vi "Placas_Foco.vi"() -> ()   [LabVIEW 2021]
uses:
  <vilib>/userDefined/High Color/IMAQdx.ctl
  <vilib>/vision/driver/NI_Vision_Acquisition_Software.lvlib
  <vilib>/vision/NI_Vision_Development_Module.lvlib
panel:
  out "String":string
  out "Matches[0].Position.y":sgl
  out "Matches[0].Position.x":sgl
  in  "Reconocer":bool
  in  "Stop":bool
  in  "Camara":T1
  out "Imagen":T2(plugin-control)
  out "Muestra":T2(plugin-control)
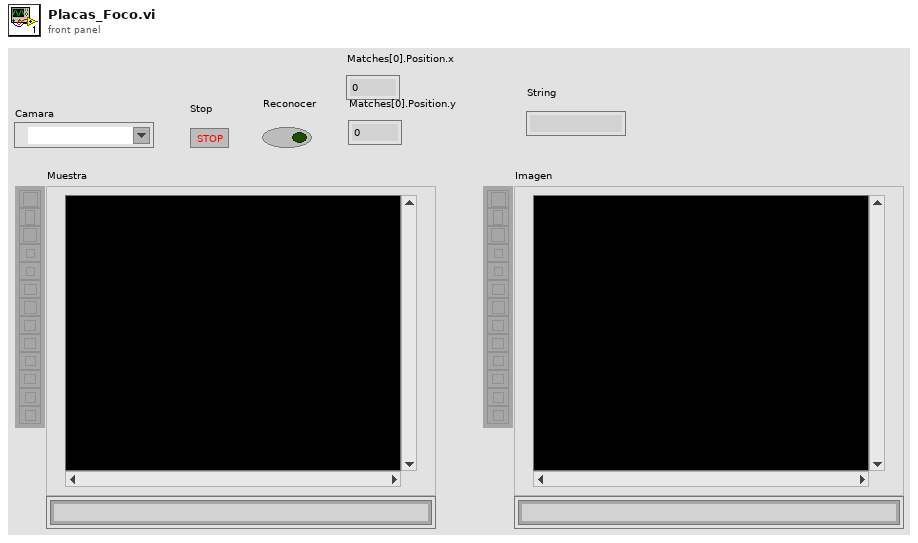
[diagram p1: front panel]
types:
  T1 = typedef "IMAQdx.ctl" = refnum<k21>
  T2 = typedef "IMAQ Image.ctl" = refnum<image>
  T3 = typedef "Image Type" = u32
  T4 = cluster{"Match Mode":u16, "Number of Matches Requested":i32, "Minimum Match Score":sgl, "SubPixel Accuracy":bool, "Rotation Angle Ranges":cluster{"Start":sgl, "End":sgl}[], "Show Search Area":bool, "Show Result":bool}
  T5 = cluster{"Position":cluster{"x":sgl, "y":sgl}, "Angle":sgl, "Scale":sgl, "Score":sgl, "Bounding Box":cluster{"x":sgl, "y":sgl}[]}[]
  T6 = cluster{"Matches[0]":cluster{"Position":cluster{"x":sgl, "y":sgl}, "Angle":sgl, "Scale":sgl, "Score":sgl, "Bounding Box":cluster{"x":sgl, "y":sgl}[]}, "Matches[1]":cluster{"Position":cluster{"x":sgl, "y":sgl}, "Angle":sgl, "Scale":sgl, "Score":sgl, "Bounding Box":cluster{"x":sgl, "y":sgl}[]}, "Matches[2]":cluster{"Position":cluster{"x":sgl, "y":sgl}, "Angle":sgl, "Scale":sgl, "Score":sgl, "Bounding Box":cluster{"x":sgl, "y":sgl}[]}, "Matches[3]":cluster{"Position":cluster{"x":sgl, "y":sgl}, "Angle":sgl, "Scale":sgl, "Score":sgl, "Bounding Box":cluster{"x":sgl, "y":sgl}[]}, "Matches[4]":cluster{"Position":cluster{"x":sgl, "y":sgl}, "Angle":sgl, "Scale":sgl, "Score":sgl, "Bounding Box":cluster{"x":sgl, "y":sgl}[]}, "Matches[5]":cluster{"Position":cluster{"x":sgl, "y":sgl}, "Angle":sgl, "Scale":sgl, "Score":sgl, "Bounding Box":cluster{"x":sgl, "y":sgl}[]}, "Matches[6]":cluster{"Position":cluster{"x":sgl, "y":sgl}, "Angle":sgl, "Scale":sgl, "Score":sgl, "Bounding Box":cluster{"x":sgl, "y":sgl}[]}, "Matches[7]":cluster{"Position":cluster{"x":sgl, "y":sgl}, "Angle":sgl, "Scale":sgl, "Score":sgl, "Bounding Box":cluster{"x":sgl, "y":sgl}[]}, "Matches[8]":cluster{"Position":cluster{"x":sgl, "y":sgl}, "Angle":sgl, "Scale":sgl, "Score":sgl, "Bounding Box":cluster{"x":sgl, "y":sgl}[]}}
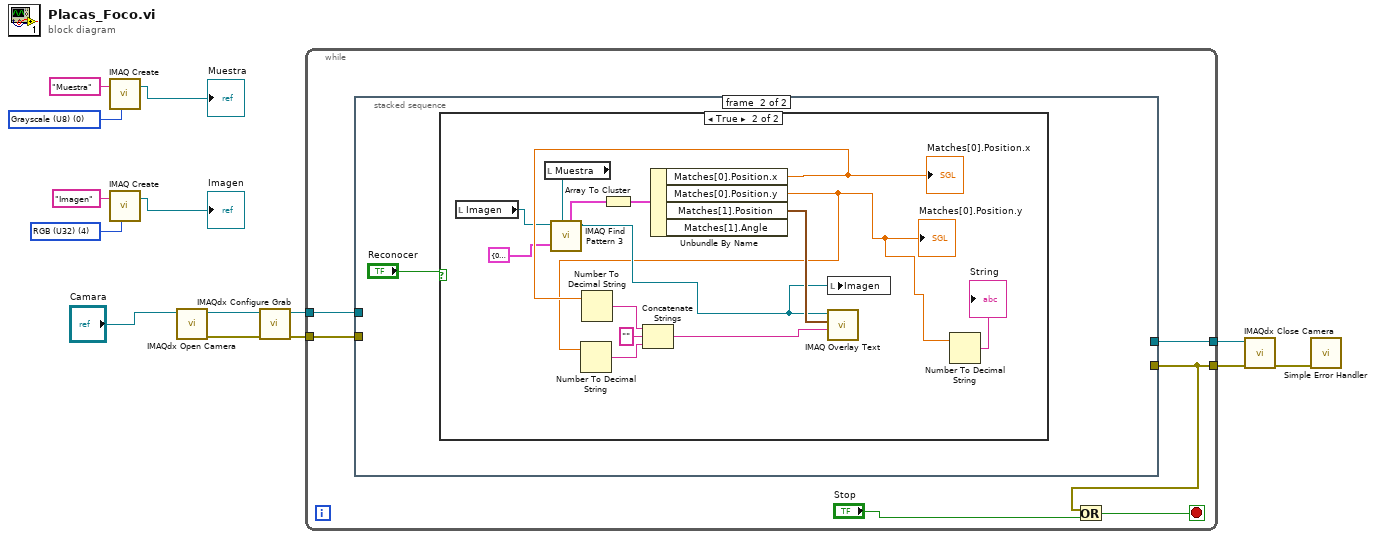
[diagram p0: block diagram]
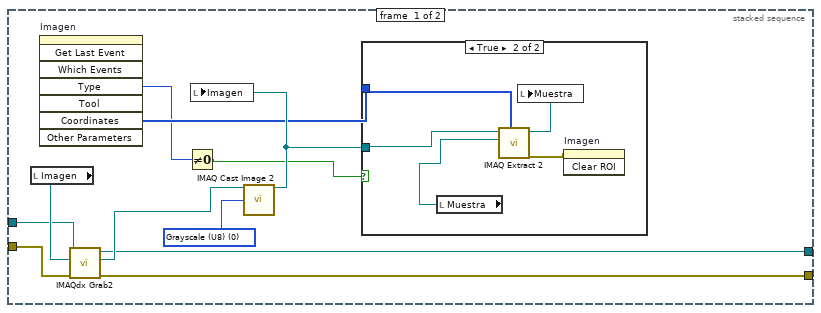
[diagram p2: hidden frame]
diagram:
  w10 = T3 4 items=["Grayscale (U8)", "Grayscale (I16)", "Grayscale (SGL)", "Complex (CSG)", "RGB (U32)", "HSL (U32)", "RGB (U64)", "Grayscale (U16)"] ("Image Type")
  w13 = T3 0 items=["Grayscale (U8)", "Grayscale (I16)", "Grayscale (SGL)", "Complex (CSG)", "RGB (U32)", "HSL (U32)", "RGB (U64)", "Grayscale (U16)"] ("Image Type")
  n1 = call "IMAQ Create"("Image Name"="Muestra", "Image Type"=w13) -> ("New Image"=→"Muestra":T2)  [unwired: 3 in, 1 out]
  n2 = call "IMAQ Create"("Image Name"="Imagen", "Image Type"=w10) -> ("New Image"=→"Imagen":T2)  [unwired: 3 in, 1 out]
  n3 = call <vilib>:"IMAQdx Open Camera.vi"("Session In"="Camara") -> ("error out"=w6:errorcluster, "Session Out"=w7:T1)  [unwired: 9 in]
  n4 = call <vilib>:"IMAQdx Configure Grab.vi"("error in"=w6, "Session In"=w7) -> ("error out"=w4:errorcluster, "Session Out"=w5:T1)  [unwired: 8 in]
  n5 = while {
    tunnel: w5 -> [w20]
    tunnel: w4 -> [w19]
    tunnel: [w18] -> w3
    tunnel: [w15] -> w2
    stop <- w17 stop-if-true
    n6 = stacked-sequence {
      tunnel: w20 -> [w30 _]
      tunnel: w19 -> [w26 _]
      tunnel: [w22 _] -> w18
      tunnel: [w21 _] -> w15
      frame #0 {
        w28 = T3 0 items=["Grayscale (U8)", "Grayscale (I16)", "Grayscale (SGL)", "Complex (CSG)", "RGB (U32)", "HSL (U32)", "RGB (U64)", "Grayscale (U16)"] ("Image Type")
        n7 = local read "Imagen"() -> (w31:T2)
        n8 = invoke on="Imagen" class="ImageControl" method="Get Last Event"() -> ("Type"=w24:i32, "Coordinates"=w25:i32[])  [unwired: 8 in, 6 out]
        n9 = call <vilib>:"IMAQdx Grab2.vi"("error in"=w26, "Image In"=w31, "Session In"=w30) -> ("error out"=w21:errorcluster, "Image Out"=w29:T2, "Session Out"=w22:T1)  [unwired: 5 in, 1 out]
        n10 = Not Equal To 0?(x=w24) -> (x != 0?=w23:bool)
        n11 = call "IMAQ Cast Image 2"("Image Src"=w29, "Image Type"=w28) -> ("Image Dst Out"=w27:T2)  [unwired: 12 in, 1 out]
        n12 = local write "Imagen"(w27) -> ()
        n13 = case shown="True" w23 {
          tunnel: w27 -> [_ w36]
          tunnel: w25 -> [_ w33]
          frame False {
          }
          frame True {
            n14 = local read "Muestra"() -> (w35:T2)
            n15 = call "IMAQ Extract 2"("Optional Rectangle"=w33, "Image Dst"=w35, "Image Src"=w36) -> ("error out"=w32:errorcluster, "Image Dst Out"=w34:T2)  [unwired: 7 in]
            n16 = local write "Muestra"(w34) -> ()
            n17 = invoke on="Imagen" class="ImageControl" method="Clear ROI"(error in=w32) -> ()  [unwired: 2 in, 3 out]
          }
        }
      }
      frame #1 {
        n18 = case shown="True" "Reconocer" {
          frame False {
          }
          frame True {
            n19 = local read "Imagen"() -> (w42:T2)
            n20 = local read "Muestra"() -> (w41:T2)
            n21 = call "IMAQ Find Pattern 3"("Settings"=T4 {"Match Mode"=0, "Number of Matches Requested"=1, "Minimum Match Score"=800.0, "SubPixel Accuracy"=FALSE, "Rotation Angle Ranges"=[], "Show Search Area"=FALSE, "Show Result"=TRUE}, "Template"=w41, "Image"=w42) -> ("Image Out"=w43:T2, "Matches"=w51:T5)  [unwired: 3 in, 4 out]
            n22 = Array To Cluster(array=w51) -> (cluster=w50:T6)
            n23 = Unbundle By Name(w50) -> ("Matches[0].Position.x"=w48:sgl, "Matches[0].Position.y"=w39:sgl, "Matches[1].Position"=w44:cluster{"x":sgl, "y":sgl})  [unwired: 1 out]
            "Matches[0].Position.x" <- w48
            "Matches[0].Position.y" <- w39
            n24 = Number To Decimal String(number=w39) -> (decimal integer string=w47:string)  [unwired: 1 in]
            n25 = Number To Decimal String(number=w48) -> (decimal integer string=w49:string)  [unwired: 1 in]
            n26 = Concatenate Strings(w49, "" ("string"), w47) -> (w45:string)
            n27 = local write "Imagen"(w43) -> ()
            n28 = call "IMAQ Overlay Text"("String"=w45, "Origin"=w44, "Image"=w43) -> ()  [unwired: 7 in, 2 out]
            n29 = Number To Decimal String(number=w39) -> (decimal integer string=→"String":string)  [unwired: 1 in]
          }
        }
      }
    }
    n30 = Or(x=w15, y="Stop") -> (x .or. y?=w17:bool)
  }
  n31 = call <vilib>:"IMAQdx Close Camera.vi"("error in"=w2, "Session In"=w3) -> ("error out"=w1:errorcluster)  [unwired: 9 in]
  n32 = call <vilib>:"Simple Error Handler.vi"("error in (no error)"=w1) -> ()  [unwired: 4 in, 5 out]
